vi "ResonanceAnalyzer.vi"() -> ()   [LabVIEW 2013]
doc: "This VI reads a spreadsheet .txt data file of the Kundt's tube and then performs a curve fit reports the RMS amplitude at resonance, the resonant frequency, and the Q factor. The VI can also simulate a data set with supplied parameters, add guassian noise and verify the fit worls correctly. This simulated data can also be used to adjust the best guess to fit parameters."
uses:
  <vilib>/imath/engines/lvmath2/RunTimeEngine/ErrorHandling/NIMS_Finalize Error.vi
  <vilib>/imath/engines/lvmath2/RunTimeEngine/Managers/WorkSpace/UID Generator.vi
  <vilib>/imath/engines/lvmath2/RunTimeEngine/Managers/SymbolTable/Clear UID.vi
  <vilib>/imath/engines/lvmath2/RunTimeEngine/NodeEndStatement/NIMS_NodeEndStatement_Output.vi
  <instcachedir>/0/NIMS_NodeEndStatement_Output_53EC0D466D134D7ABD903AC30B43404B.lvgen/NIMS_NodeEndStatement_Output_53EC0D466D134D7ABD903AC30B43404B_005.vi
  <instcachedir>/0/NIMS_NodeEndStatement_Output_53EC0D466D134D7ABD903AC30B43404B.lvgen/NIMS_NodeEndStatement_Output_53EC0D466D134D7ABD903AC30B43404B_000.vi
  <vilib>/imath/engines/lvmath2/RunTimeEngine/RangeToken/NIMS_Range.vi
  <instcachedir>/0/NIMS_Range_CC84A22A7D615C41BA1124D7A0F122CE.lvgen/NIMS_Range_CC84A22A7D615C41BA1124D7A0F122CE_000.vi
  <vilib>/imath/engines/lvmath2/RunTimeEngine/RunTimeType/NIMS_RunTimeType_From StrictType (excl LVString).vi
  <instcachedir>/0/NIMS_RunTimeType_From StrictType (excl LVString)_57CF553C4D5778428DA95AEC531EE8B5.lvgen/NIMS_RunTimeType_From StrictType (excl LVString)_57CF553C4D5778428DA95AEC531EE8B5_000.vi
  <vilib>/imath/engines/lvmath2/RunTimeEngine/LocalVariableDefStatement/MC_LocalVariableDefStatement_Display.vi
  <vilib>/imathl/engines/lvmath/Functions/Error Handling/Create Error.vi
  <vilib>/imath/engines/lvmath2/RunTimeEngine/BuiltInFunctions/randnormal/NIMS_randnormal(1,I32).vi
  <vilib>/imath/engines/lvmath2/RunTimeEngine/ErrorHandling/NIMS_Error From Error Code.vi
  <vilib>/imath/engines/lvmath2/RunTimeEngine/ArithmeticOperatorToken/NIMS_ArithmeticOperator_minus.vi
  <instcachedir>/0/NIMS_ArithmeticOperator_minus_0CB5619037AD224A984EE9CC97976825.lvgen/NIMS_ArithmeticOperator_minus_0CB5619037AD224A984EE9CC97976825_003.vi
  <vilib>/imath/engines/lvmath2/RunTimeEngine/ArithmeticOperatorToken/NIMS_ArithmeticOperator_plus.vi
  <instcachedir>/0/NIMS_ArithmeticOperator_plus_AEA2D963A4FCCF419CCDFE3DED9E11BA.lvgen/NIMS_ArithmeticOperator_plus_AEA2D963A4FCCF419CCDFE3DED9E11BA_001.vi
  <vilib>/Utility/file.llb/Read From Spreadsheet File (DBL).vi
  <vilib>/imath/engines/lvmath2/RunTimeEngine/Managers/SymbolTable/NIMS_WorkSpace.lvlib
panel:
  out "XY Graph":cluster{"f":dbl[], "y":dbl[]}[](graph)=[{"f"=[600.0, 601.0, 602.0, 602.0, 603.0, 604.0, 604.0, 605.0, 606.0, 607.0, 608.0, 608.0, 609.0, 610.0, 610.0, 611.0, 612.0, 613.0, 614.0, 614.0, 615.0, 616.0, 616.0, 617.0, 618.0, 619.0, 620.0, 620.0, 621.0, 622.0, 622.0, 623.0, 624.0, 625.0, 626.0, 626.0, 627.0, 628.0, 628.0, 629.0, 630.0, 631.0, 632.0, 632.0, 633.0, 634.0, 634.0, 635.0, 636.0, 637.0, 638.0, 638.0, 639.0, 640.0, 640.0, 641.0, 642.0, 643.0, 644.0, 644.0, 645.0, 646.0, 646.0, 647.0, 648.0, 649.0, 650.0, 650.0, 651.0, 652.0, 652.0, 653.0, 654.0, 655.0, 656.0, 656.0, 657.0, 658.0, 658.0, 659.0, 660.0, 661.0, 662.0, 662.0, 663.0, 664.0, 664.0, 665.0, 666.0, 667.0, 668.0, 668.0, 669.0, 670.0, 670.0, 671.0, 672.0, 673.0, 674.0, 674.0, 675.0, 676.0, 676.0, 677.0, 678.0, 679.0, 680.0, 680.0, 681.0, 682.0, 682.0, 683.0, 684.0, 685.0, 686.0, 686.0, 687.0, 688.0, 688.0, 689.0, 690.0, 691.0, 692.0, 692.0, 693.0, 694.0, 694.0, 695.0, 696.0, 697.0, 698.0, 698.0, 699.0, 700.0, 700.0, 701.0, 702.0, 703.0, 704.0, 704.0, 705.0, 706.0, 706.0, 707.0, 708.0, 709.0, 710.0, 710.0, 711.0, 712.0, 712.0, 713.0, 714.0, 715.0, 716.0, 716.0, 717.0, 718.0, 718.0, 719.0, 720.0, 721.0, 722.0, 722.0, 723.0, 724.0, 724.0, 725.0, 726.0, 727.0, 728.0, 728.0, 729.0, 730.0, 730.0, 731.0, 732.0, 733.0, 734.0, 734.0, 735.0, 736.0, 736.0, 737.0, 738.0, 739.0, 740.0, 740.0, 741.0, 742.0, 742.0, 743.0, 744.0, 745.0, 746.0, 746.0, 747.0, 748.0, 748.0, 749.0, 750.0], "y"=[0.1432352795490912, 0.13840443284038806, 0.13854791675667233, 0.13999096265683428, 0.13995873225726185, 0.14135136280792865, 0.14247871840593188, 0.14261000660632964, 0.1437639510712277, 0.14491054840012255, 0.14672360869077516, 0.147842739040067, 0.1478938109324158, 0.1494169957406701, 0.15114716300850065, 0.15106018074531244, 0.15323218697307633, 0.15486383150737476, 0.15700012565614901, 0.15909260753402207, 0.15909260753402207, 0.1613986879824255, 0.16793839566345561, 0.16375704768835847, 0.16672472125510626, 0.1691609050277635, 0.17204814718780956, 0.1752871177601893, 0.17482357622374528, 0.17786889211498957, 0.18144708686925964, 0.18119658153762153, 0.18471407949096041, 0.1882781836734676, 0.19219850268883043, 0.1962682273314004, 0.19635863300537473, 0.20051644670498045, 0.20495098033339565, 0.20511621788255657, 0.21081426762531869, 0.21574960039467433, 0.2205464136392749, 0.22622989815726405, 0.22633410486812164, 0.23278232416822928, 0.23919384495683124, 0.23894612943407997, 0.2460650880742456, 0.25351286304979076, 0.2618484455029599, 0.2703958364108844, 0.2705203869719352, 0.27983369045620216, 0.29046914073819097, 0.29000133690540686, 0.3006768556972182, 0.3126079367123955, 0.3257991898248433, 0.33892218687275544, 0.33950799043200497, 0.3545275586178804, 0.37051005630192396, 0.37089416418640336, 0.3888212570527512, 0.40850746766312496, 0.43008074565603494, 0.45368038204688277, 0.4539938816187383, 0.4800096849081116, 0.5086862516043105, 0.5085105879351045, 0.5391380704697852, 0.5732578361071086, 0.6084151222917087, 0.6465468497750434, 0.6464724176028751, 0.6849360107591052, 0.7211074791828996, 0.7220212839244983, 0.755440040567619, 0.7845127388202923, 0.8059349691127455, 0.8169585080397148, 0.8169585080397148, 0.815361122738876, 0.8014012214056273, 0.8014934914423114, 0.7769623959921387, 0.7441320326267459, 0.7068056297002477, 0.6669603248243565, 0.6674212038584768, 0.6274079248328789, 0.5887080847020436, 0.588843655355589, 0.5536687348429373, 0.5190390101970822, 0.48842737842292505, 0.45956823187215834, 0.46015060778905875, 0.4344602022128757, 0.4102513321979177, 0.41077121255338767, 0.3890003570949605, 0.369530253547673, 0.3516009177497919, 0.33535130445056066, 0.3351969050221628, 0.32029488265137857, 0.30630211810503166, 0.3064432079278907, 0.2936635198916893, 0.28190319626364724, 0.27114400086883106, 0.2615471548094848, 0.26127628960311017, 0.2524933822964291, 0.24350057999520247, 0.24296851537593975, 0.23536939986722874, 0.22821805513022142, 0.22102937721758537, 0.21414108558785827, 0.21473359748208543, 0.20840109665884488, 0.20241840573760617, 0.20239510279887693, 0.19672067232252666, 0.19191105813411904, 0.18702514494718114, 0.18270481798956184, 0.18251560400913677, 0.17844319885403656, 0.17410049263526076, 0.1739802698038288, 0.17076544728138743, 0.16649454157952753, 0.16328639466631975, 0.16037992276693455, 0.1603614594088224, 0.15694590909721592, 0.15390403281864123, 0.15378005078810528, 0.1514607140703406, 0.1487989956986022, 0.14574712612565288, 0.1439792808458691, 0.14378050346057386, 0.14203651240480114, 0.13954041170406153, 0.13966899237730424, 0.1368831529074947, 0.13545654682426905, 0.13350575895623717, 0.13164367570556065, 0.13144679457894223, 0.13016673155792644, 0.1284547002378748, 0.12860267434121764, 0.12683817950005424, 0.1257476854367659, 0.1236516739349173, 0.12230663002323712, 0.12240523724999103, 0.12181478415073504, 0.1199775529871384, 0.1199637408559937, 0.11920651731327471, 0.11793697928023808, 0.11664066848842987, 0.11591776527998855, 0.11649304569904531, 0.11519934240465526, 0.11410377163197279, 0.11460405911366027, 0.11363182976673103, 0.11274570328651795, 0.11226645259802344, 0.1115835052288668, 0.11126280383196824, 0.11050959823315383, 0.11003985260653876, 0.1098752813118071, 0.10960995513841977, 0.10909378253153822, 0.10853004922771126, 0.10795679926883704, 0.1081433951297938, 0.10824304476091305, 0.1076465213629835, 0.10726301496168973, 0.10711492794856042, 0.1069916782922137, 0.10670874200130985, 0.10636530750764384, 0.1064020511283989, 0.10632857657549442, 0.10615733320165413, 0.10630409633445627, 0.10613289238632076]}, ...(2 in all)]
  out "Center Frequency":dbl=662.7362583608757
  out "Q Factor":dbl=38.53052738463516
  out "Amplitude":dbl=0.8051212727852404
  in  "?":enum32{"Sim", "Data"}(tab)=enum."Data"
  in  "Input Parameters":T1={"Q Factor"=10.0, "Center Frequency"=600.0, "Start Frequency"=400.0, "End Frequency"=800.0, "dF"=5.0, "Noise Level"=0.01, "RMS Voltage Amplitude"=2.0}
  # "Will curve fit data from a spreadsheet\n.txt file"
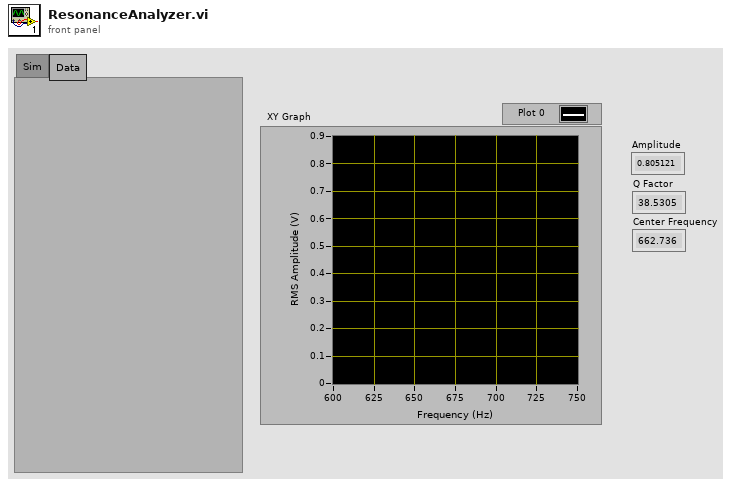
[diagram p1: front panel]
types:
  T1 = cluster{"Q Factor":dbl, "Center Frequency":dbl, "Start Frequency":dbl, "End Frequency":dbl, "dF":dbl, "Noise Level":dbl, "RMS Voltage Amplitude":dbl}
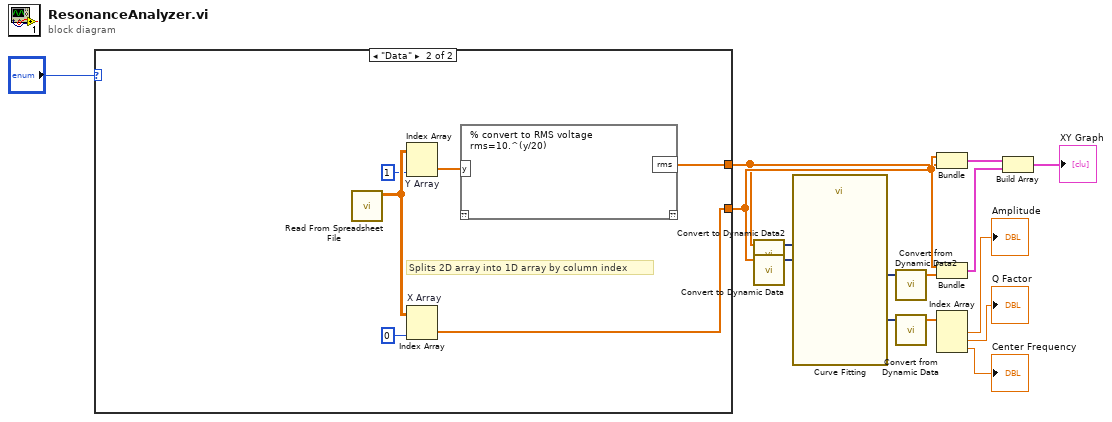
[diagram p0: block diagram]
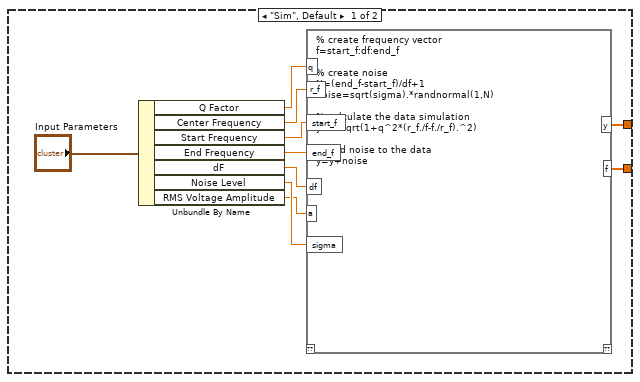
[diagram p2: hidden frame]
diagram:
  n1 = case shown="\"Data\"" "?" {
    tunnel: [w18 w200] -> w4
    tunnel: [w19 w201] -> w14
    frame "Sim", Default {
      n2 = Unbundle By Name("Input Parameters") -> ("Q Factor"=w24:dbl, "Center Frequency"=w23:dbl, "Start Frequency"=w22:dbl, "End Frequency"=w21:dbl, "dF"=w20:dbl, "Noise Level"=w17:dbl, "RMS Voltage Amplitude"=w16:dbl)
      n3 = mathscript code="% create frequency vector\nf=start_f:df:end_f\n\n% create noise\nN=(end_f-start_f)/df+1\nnoise=sqrt(sigma).*randnormal(1,N)\n\n% calculate the data simulation\ny=a./sqrt(1+q^2*(r_f./f-f./r_f).^2)\n\n% add noise to the data\ny=y+noise"("q"=w24, "r_f"=w23, "a"=w16, "df"=w20, "start_f"=w22, "end_f"=w21, "sigma"=w17) -> ("y"=w18:cdb[], "f"=w19:dbl[])  [unwired: 1 in, 1 out]
    }
    frame "Data" {
      # "Splits 2D array into 1D array by column index"
      n4 = call-poly <vilib>:"Read From Spreadsheet File.vi"() -> ("all rows"=w204:dbl[][])  [unwired: 7 in, 4 out]
      n5 = Index Array "Y Array"(array=w204, index (col)=1 ("disabled index (col)")) -> (element=w199:dbl[])  [unwired: 1 in]
      n6 = Index Array "X Array"(array=w204, index (col)=0 ("disabled index (col)")) -> (element=w201:dbl[])  [unwired: 1 in]
      n7 = mathscript code="% convert to RMS voltage\nrms=10.^(y/20)"("y"=w199) -> ("rms"=w200:dbl[])  [unwired: 1 in, 1 out]
    }
  }
  n8 = call "Convert to Dynamic Data2"("Array"=w4) -> ("Dynamic Data Type"=w12:dynamicdata)  [unwired: 3 in]
  n9 = call "Convert to Dynamic Data"("Array"=w14) -> ("Dynamic Data Type"=w13:dynamicdata)  [unwired: 3 in]
  n10 = call "Curve Fitting"("Locations"=w13, "Signals"=w12) -> ("best fit"=w6:dynamicdata, "non-linear coefficients"=w11:dynamicdata)  [unwired: 5 in, 3 out]
  n11 = call "Convert from Dynamic Data2"("Dynamic Data Type"=w6) -> ("Array"=w5:dbl[])  [unwired: 3 in]
  n12 = call "Convert from Dynamic Data"("Dynamic Data Type"=w11) -> ("Array"=w10:dbl[])  [unwired: 3 in]
  n13 = Bundle("all rows"=w14, "y"=w4) -> (w2:cluster{"all rows":dbl[], "y":cdb[]})  [unwired: 1 in]
  n14 = Bundle("all rows"=w14, "Array"=w5) -> (w3:cluster{"all rows":dbl[], "Array":dbl[]})  [unwired: 1 in]
  n15 = Index Array(array=w10) -> (element #1=→"Amplitude":dbl, element #2=→"Q Factor":dbl, element #3=→"Center Frequency":dbl)  [unwired: 3 in]
  n16 = Build Array(w2, w3) -> (→"XY Graph":cluster{"all rows":dbl[], "y":cdb[]}[])
